vi "Rcv_Cmd_uncorrupted.vi"(8 "error in (no error)":errorcluster, 11 "cPAS in":refnum<class "cPAS.lvclass">) -> (0 "error out":errorcluster, 3 "cPAS out":refnum<class "cPAS.lvclass">)   [LabVIEW 2015, in "cPAS.lvclass"]
uses:
  cPAS.lvclass
  Reusable/Instrument/state.ctl
  Reusable/Instrument/Instrument.lvclass
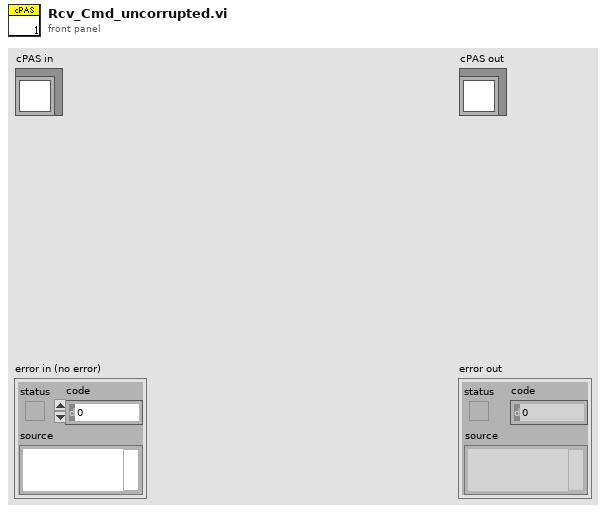
[diagram p1: front panel]
types:
  T1 = typedef "Instrument.lvclass/state.ctl" = enum8{"Configure", "Acquire", "Wait", "Quit", "Handle Error", "NOOP"}
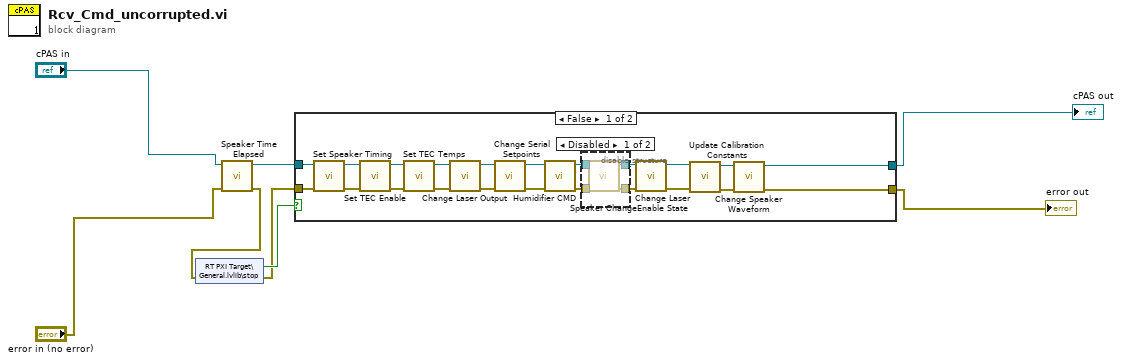
[diagram p0: block diagram]
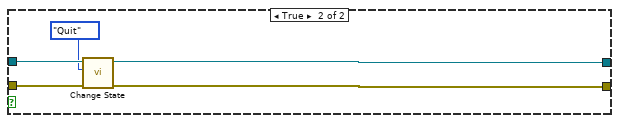
[diagram p3: hidden frame]
diagram:
  n1 = call-dynamic "Speaker Time Elapsed.vi"("error in"="error in (no error)", "cPAS in"="cPAS in") -> ("error out"=w3:errorcluster, "cPAS out"=w6:refnum<class "cPAS.lvclass">)  [unwired: 7 in, 1 out]
  n2 = shared-variable "RT PXI Target\\General.lvlib\\stop"(error in=w3) -> (w8:bool, error out=w7:errorcluster)
  n3 = case shown="False" w8 {
    tunnel: w6 -> [w30 w41]
    tunnel: w7 -> [w29 w38]
    tunnel: [w10 w39] -> w1
    tunnel: [w9 w37] -> w2
    frame False {
      n4 = call-dynamic "Set Speaker Timing.vi"("error in"=w29, "cPAS in"=w30) -> ("error out"=w22:errorcluster, "cPAS out"=w20:refnum<class "cPAS.lvclass">)  [unwired: 8 in]
      n5 = call-dynamic "Set TEC Enable.vi"("error in"=w22, "cPAS in"=w20) -> ("error out"=w21:errorcluster, "cPAS out"=w19:refnum<class "cPAS.lvclass">)  [unwired: 8 in]
      n6 = call-dynamic "Set TEC Temps.vi"("error in"=w21, "cPAS in"=w19) -> ("error out"=w26:errorcluster, "cPAS out"=w24:refnum<class "cPAS.lvclass">)  [unwired: 8 in]
      n7 = call-dynamic "Change Laser Output.vi"("error in"=w26, "cPAS in"=w24) -> ("error out"=w25:errorcluster, "cPAS out"=w23:refnum<class "cPAS.lvclass">)  [unwired: 8 in]
      n8 = call "Change Serial Setpoints.vi"("error in"=w25, "cPAS in"=w23) -> ("error out"=w27:errorcluster, "cPAS out"=w28:refnum<class "cPAS.lvclass">)  [unwired: 8 in]
      n9 = call "Humidifier CMD.vi"("error in"=w27, "cPAS in"=w28) -> ("error out"=w17:errorcluster, "cPAS out"=w18:refnum<class "cPAS.lvclass">)  [unwired: 8 in]
      n10 = disable-structure shown="Disabled" {
        disable-tunnel: w18 -> [w34 w36]
        disable-tunnel: w17 -> [w33 w35]
        disable-tunnel: [w32 w36] -> w16
        disable-tunnel: [w31 w35] -> w15
        frame Disabled {
          n11 = call "Speaker Change.vi"("error in"=w33, "cPAS in"=w34) -> ("error out"=w31:errorcluster, "cPAS out"=w32:refnum<class "cPAS.lvclass">)  [unwired: 8 in]
        }
        frame Enabled {
        }
      }
      n12 = call "Change Laser Enable State.vi"("error in"=w15, "cPAS in"=w16) -> ("error out"=w13:errorcluster, "cPAS out"=w14:refnum<class "cPAS.lvclass">)  [unwired: 8 in]
      n13 = call "Update Calibration Constants.vi"("error in"=w13, "cPAS in"=w14) -> ("error out"=w11:errorcluster, "cPAS out"=w12:refnum<class "cPAS.lvclass">)  [unwired: 8 in]
      n14 = call "Change Speaker Waveform.vi"("error in"=w11, "cPAS in"=w12) -> ("error out"=w9:errorcluster, "cPAS out"=w10:refnum<class "cPAS.lvclass">)  [unwired: 8 in]
    }
    frame True {
      n15 = call "Change State.vi"("error in"=w38, "instr state"=state."Quit", "Instrument in"=w41) -> ("error out"=w37:errorcluster, "Instrument out"=w39:refnum<class "cPAS.lvclass">)  [unwired: 7 in]
    }
  }
  "error out" <- w2
  "cPAS out" <- w1
